vi "rqcBob Check Status.vi"(0 "rqcBob in":refnum<class "rqcBob.lvclass">, 11 "error in (no error)":errorcluster) -> (4 "rqcBob out":refnum<class "rqcBob.lvclass">, 6 "done?":bool, 15 "error out":errorcluster)   [LabVIEW 2019, in "rqcBob.lvclass"]
uses:
  rqcBob.lvclass
  rqcBob.lvclass/rqcBob.ctl
  Custom Controls/rqcBob Main FPGA interface.ctl
  <vilib>/Utility/error.llb/Error Cluster From Error Code.vi
  <vilib>/rvi/errors/niLvFpgaAdjustHostInterfaceError.vi
  <vilib>/rvi/interface/nirviReadWriteControl/nirviReadWriteControl.xnode
  NiFpgaLv.dll
  <vilib>/rvi/interface/Simulation/niFpgaSimulationCallBeginRW.vi
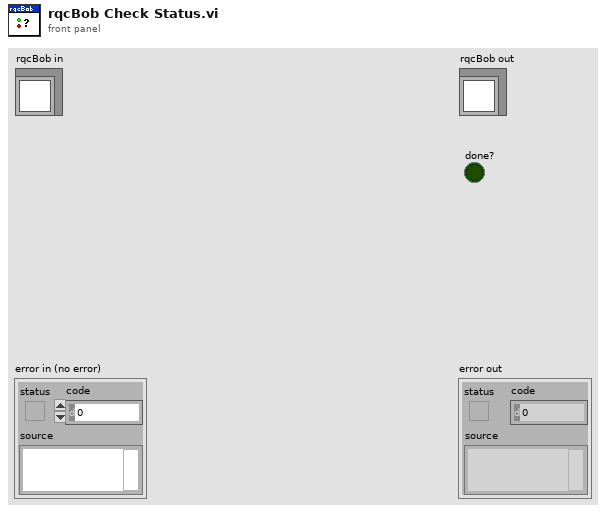
[diagram p1: front panel]
types:
  T1 = typedef "rqcBob.lvclass/rqcBob Main FPGA interface.ctl" = refnum<k20>
  T2 = typedef "rqcBob.lvclass/rqcBob State.ctl" = enum16{"Idle", "Run"}
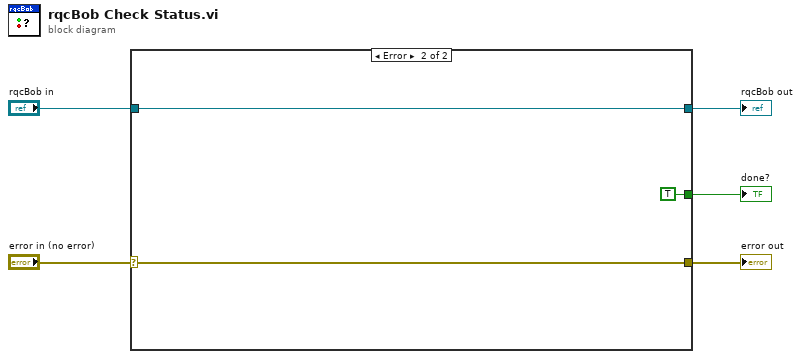
[diagram p0: block diagram]
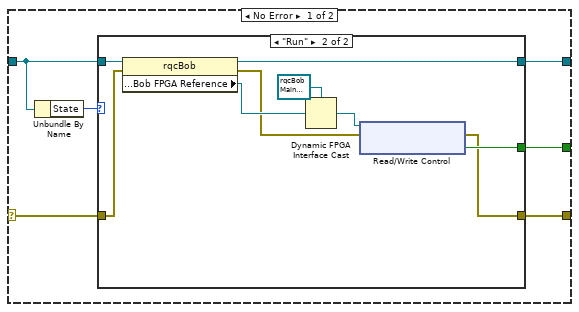
[diagram p2: hidden frame]
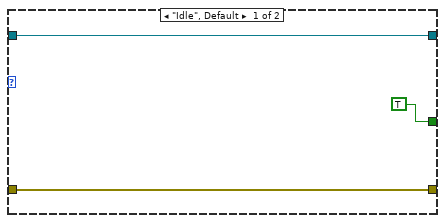
[diagram p3: hidden frame]
diagram:
  n1 = case shown="Error" "error in (no error)" {
    selector: "error in (no error)" -> [w7 w26]
    tunnel: [w6 w26] -> w4
    tunnel: [w8 w25] -> w2
    tunnel: "rqcBob in" -> [w9 w25]
    tunnel: [w10 TRUE] -> w1
    frame No Error {
      n2 = Unbundle By Name(w9) -> ("State"=w11:T2)
      n3 = case shown="\"Run\"" w11 {
        tunnel: [TRUE w16] -> w10
        tunnel: w9 -> [w13 w21]
        tunnel: [w13 w20] -> w8
        tunnel: [w12 w15] -> w6
        tunnel: w7 -> [w12 w19]
        frame "Idle", Default {
        }
        frame "Run" {
          n4 = property class="rqcBob"(reference=w21, error in=w19) -> (reference out=w20:refnum<class "rqcBob.lvclass">, error out=w17:errorcluster, "public:Public Properties Access:Bob FPGA Reference"=w22:refnum<k20>)
          n5 = Dynamic FPGA Interface Cast(Session In=T1 refnum ("Bob main FPGA interface"), Type=w22) -> (Session Out=w18:T1)
          n6 = xnode "Read/Write Control"("FPGA VI Reference In"=w18, "error in"=w17) -> ("error out"=w15:errorcluster, "generation.done"=w16:bool)  [unwired: 1 out]
        }
      }
    }
    frame Error {
    }
  }
  "error out" <- w4
  "rqcBob out" <- w2
  "done?" <- w1
